vi "Read UI References.vi"(8 "error in (no error)":errorcluster, 11 "Results in":refnum<class "Results.lvclass">) -> (0 "error out":errorcluster, 2 "UI References":T1, 3 "Results out":refnum<class "Results.lvclass">)   [LabVIEW 2017, in "Result Actor.lvlib" / "Results.lvclass"]
uses:
  Results.lvclass
  UI References.ctl
  Results.lvclass/Results.ctl
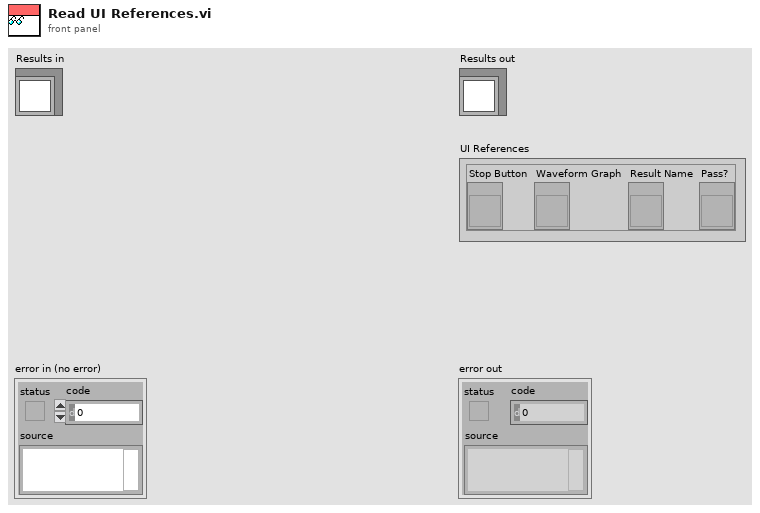
[diagram p1: front panel]
types:
  T1 = typedef "Result Actor.lvlib/Results.lvclass/UI References.ctl" = cluster{"Stop Button":refnum<vi>, "Waveform Graph":refnum<vi>, "Result Name":refnum<vi>, "Pass?":refnum<vi>}
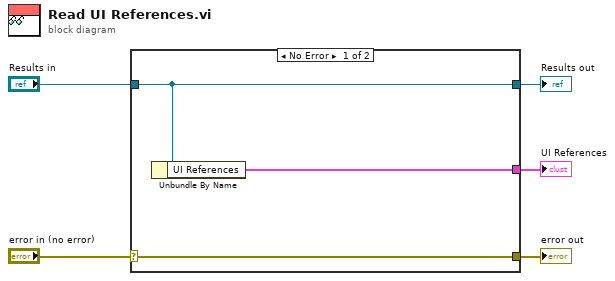
[diagram p0: block diagram]
diagram:
  n1 = case shown="No Error" "error in (no error)" {
    selector: "error in (no error)" -> [w8 w9]
    tunnel: [w8 w9] -> w4
    tunnel: [w7 w10] -> w2
    tunnel: "Results in" -> [w7 w10]
    tunnel: [w6 _] -> w1
    frame No Error {
      n2 = Unbundle By Name(w7) -> ("UI References"=w6:T1)
    }
    frame Error {
    }
  }
  "error out" <- w4
  "Results out" <- w2
  "UI References" <- w1
